vi "handle_ALP_error.vi"(8 "error in":errorcluster, 11 "Return Codes":i32[](array[numeric])) -> (0 "error out":errorcluster)   [LabVIEW 2020]
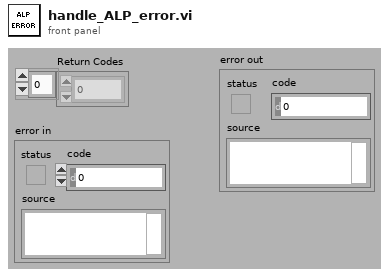
[diagram p1: front panel]
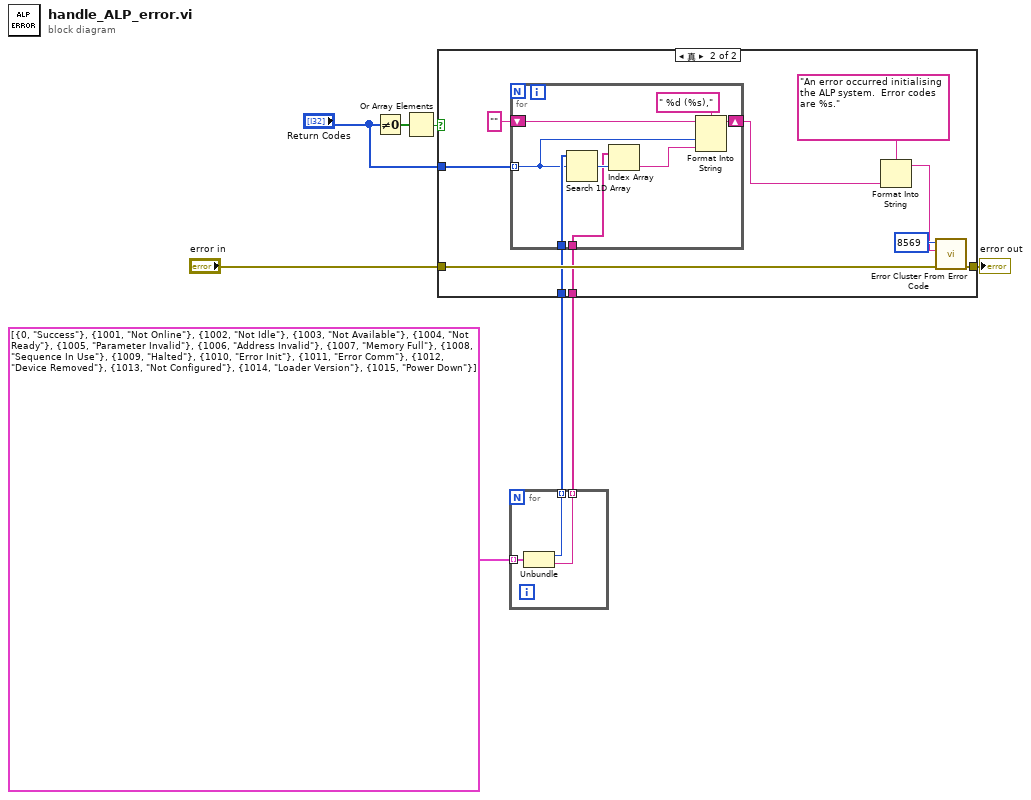
[diagram p0: block diagram]
diagram:
  n1 = Not Equal To 0?(x="Return Codes") -> (x != 0?=w4:bool[])
  n2 = Or Array Elements(Boolean array=w4) -> (logical OR=w7:bool)
  n3 = for {
    tunnel: cluster{i32, string}[] [{0, "Success"}, {1001, "Not Online"}, {1002, "Not Idle"}, {1003, "Not Available"}, {1004, "Not Ready"}, {1005, "Parameter Invalid"}, {1006, "Address Invalid"}, {1007, "Memory Full"}, {1008, "Sequence In Use"}, {1009, "Halted"}, {1010, "Error Init"}, {1011, "Error Comm"}, {1012, "Device Removed"}, {1013, "Not Configured"}, {1014, "Loader Version"}, {1015, "Power Down"}] -> [w11] mode=indexing
    tunnel: [w10] -> w2 mode=indexing
    tunnel: [w9] -> w1 mode=indexing
    n4 = Unbundle(w11) -> (w10:i32, w9:string)
  }
  n5 = case shown="真" w7 {
    tunnel: "error in" -> [w12 w22]
    tunnel: [w12 w21] -> w6
    tunnel: "Return Codes" -> [_ w17]
    tunnel: w2 -> [_ w16]
    tunnel: w1 -> [_ w15]
    frame False {
    }
    frame True {
      n6 = for {
        tunnel: w17 -> [w26] mode=indexing
        tunnel: w16 -> [w30]
        tunnel: w15 -> [w28]
        shift-right: [w24] -> w13
        shift-left: "" -> [w23]
        n7 = Search 1D Array(1D array=w30, element=w26) -> (index of element=w29:i32)  [unwired: 1 in]
        n8 = Index Array(array=w28, index=w29) -> (element=w25:string)
        n9 = Format Into String(format string=" %d (%s),", initial string=w23, w26, w25) -> (resulting string=w24:string)  [unwired: 1 in, 1 out]
      }
      n10 = Format Into String(format string="An error occurred initialising the ALP system.  Error codes are %s.", w13) -> (resulting string=w18:string)  [unwired: 2 in, 1 out]
      n11 = call <vilib>:"Error Cluster From Error Code.vi"("error in (no error)"=w22, "error message (\"\")"=w18, "error code (0)"=8569) -> ("error out"=w21:errorcluster)  [unwired: 6 in]
    }
  }
  "error out" <- w6
